vi "Bind RPC example_SignalGeneratorService_GetAnalyzedParameters.vi"(11 "gRPCid server in":T3) -> (0 "error out":errorcluster, 1 "example_SignalGeneratorService_GetAnalyzedParameters Internal UE":T2, 2 "example_SignalGeneratorService_GetAnalyzedParameters gRPC UE":T1, 3 "gRPCid server out":T3)   [LabVIEW 2019, in "NW and PSD_server.lvlib" / "NW and PSD_server.lvclass"]
uses:
  NW and PSD_server.lvclass
  <vilib>/gRPC/LabVIEW gRPC Library/Server API/typeDefs/grpcId.ctl
  typeDefs/Server Internal Message UE.ctl
  typeDefs/Server Internal Message.ctl
  <vilib>/gRPC/LabVIEW gRPC Library/Server API/typeDefs/gRPCId Cluster UE.ctl
  <vilib>/gRPC/LabVIEW gRPC Library/Server API/typeDefs/gRPCId Cluster.ctl
  616620f9-6bbe-466a-af51-04bcc3596ea0.vi
  <vilib>/gRPC/LabVIEW gRPC Library/Server API/Server/Get Server DLL Path.vi
  <vilib>/gRPC/LabVIEW gRPC Library/gprc-lvsupport-release.lvlib
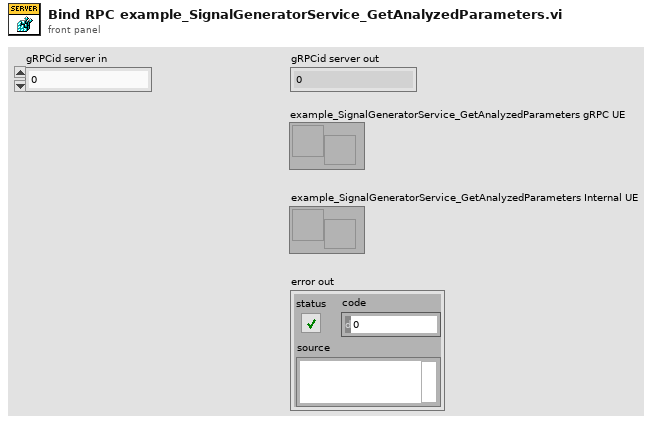
[diagram p1: front panel]
types:
  T1 = typedef "gprc-lvsupport-release.lvlib/gRPCId Cluster UE.ctl" = refnum<user-event>
  T2 = typedef "NW and PSD_server.lvlib/NW and PSD_server.lvclass/Server Internal Message UE.ctl" = refnum<user-event>
  T3 = typedef "gprc-lvsupport-release.lvlib/grpcId.ctl" = u64
  T4 = typedef "NW and PSD_server.lvlib/NW and PSD_server.lvclass/Server Internal Message.ctl" = cluster{"Command":string, "Data":variant}
  T5 = typedef "gprc-lvsupport-release.lvlib/gRPCId Cluster.ctl" = cluster{"gRPCid":T3}
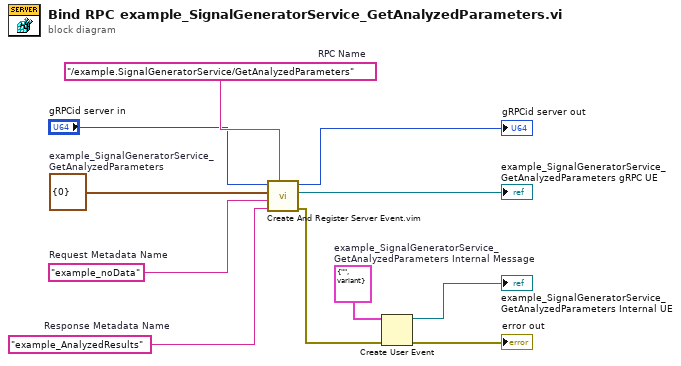
[diagram p0: block diagram]
diagram:
  w5 = T4 {"Command"="", "Data"=variant}  # example_SignalGeneratorService_GetAnalyzedParameters Internal Message
  w8 = "example_AnalyzedResults"  # Response Metadata Name
  w11 = T5 {"gRPCid"=0}  # example_SignalGeneratorService_GetAnalyzedParameters
  w9 = "example_noData"  # Request Metadata Name
  w10 = "/example.SignalGeneratorService/GetAnalyzedParameters"  # RPC Name
  n1 = call "Create And Register Server Event.vim"("Method name"=w10, "Response Metadata Name"=w8, "Request Metadata Name"=w9, "event in"=w11, "gRPCid server in"="gRPCid server in") -> ("error out"=w4:errorcluster, "event"=→"example_SignalGeneratorService_GetAnalyzedParameters gRPC UE":refnum<user-event>, "gRPCid server out"=→"gRPCid server out":T3)  [unwired: 4 in]
  n2 = Create User Event(user event datatype=w5, error in=w4) -> (user event=→"example_SignalGeneratorService_GetAnalyzedParameters Internal UE":refnum<user-event>, error out=→"error out":errorcluster)
